vi "SignalReceiverCreat.vi"() -> (14 "SignalReceiver out":refnum<class "SignalReceiver.lvclass">, 15 "事件注册引用句柄":refnum<event-registration>, 19 "错误输出":errorcluster)   [LabVIEW 2020, in "ECU_Diagnose.lvlib" / "SignalReceiver.lvclass"]
uses:
  SignalReceiver.lvclass
  C:/Program Files (x86)/National Instruments/LabVIEW 2020/vi.lib/JKI/JKI SMO/SMO/SMO.lvclass
  Typedefs/PublicEvents--Cluster.ctl
  Typedefs/SetpointChanged--EventData--Cluster.ctl
  Typedefs/Data.ctl
  <vilib>/JKI/JKI SMO/SMO/Typedefs/Public Events.ctl
  <vilib>/JKI/JKI SMO/SMO/Typedefs/SMOState --Enum.ctl
  <vilib>/JKI/JKI SMO/SMO/Typedefs/Reserve State--Enum.ctl
  <vilib>/JKI/JKI SMO/SMO/SMO.lvclass/SMO.ctl
  <vilib>/JKI/JKI SMO/SMO/Private/ReftoDVR--SMO.vi
  <vilib>/JKI/JKI SMO/SMO/SMO.lvclass
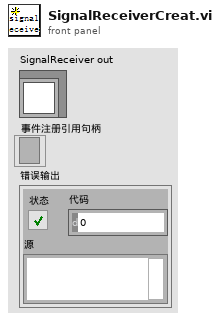
[diagram p1: front panel]
types:
  T1 = typedef "ECU_Diagnose.lvlib/SignalReceiver.lvclass/SignalArrySelecte.ctl" = cluster{"Port_No.":refnum<k21>, "XNET Signal":refnum<k21>[]}
  T2 = typedef "SMO.lvclass/Public Events.ctl" = cluster{"Error":refnum<user-event>, "State":refnum<user-event>, "Reserve State":refnum<user-event>}
  T3 = typedef "ECU_Diagnose.lvlib/SignalReceiver.lvclass/PublicEvents--Cluster.ctl" = cluster{"Setpoint Changed":refnum<user-event>, "Value Changed":refnum<user-event>}
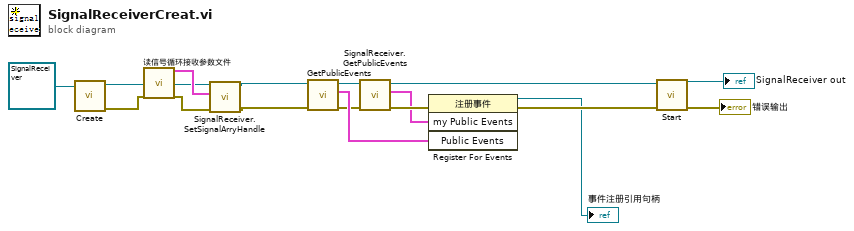
[diagram p0: block diagram]
diagram:
  n1 = call <vilib>:"Create.vi"("SMO"=refnum<class "SignalReceiver.lvclass"> refnum ("SMO.Template.lvclass")) -> ("error out"=w2:errorcluster, "SMO out"=w15:refnum<class "SignalReceiver.lvclass">)  [unwired: 8 in, 1 out]
  n2 = call "读信号循环接收参数文件.vi"("error in (no error)"=w2) -> ("SignalArryOut"=w17:T1, "error out"=w1:errorcluster)  [unwired: 17 in]
  n3 = call "SignalReceiver.SetSignalArryHandle.vi"("error in (no error)"=w1, "SignalArrySelect"=w17, "SignalReceiver"=w15) -> ("error out"=w16:errorcluster, "SignalReceiver out"=w8:refnum<class "SignalReceiver.lvclass">)  [unwired: 7 in]
  n4 = call <vilib>:"GetPublicEvents.vi"("error in (no error)"=w16, "SMO"=w8) -> ("error out"=w11:errorcluster, "Public Events"=w14:T2, "SMO out"=w12:refnum<class "SignalReceiver.lvclass">)  [unwired: 7 in]
  n5 = call "SignalReceiver.GetPublicEvents.vi"("error in (no error)"=w11, "SignalReceiver"=w12) -> ("error out"=w13:errorcluster, "my Public Events"=w10:T3, "SignalReceiver out"=w7:refnum<class "SignalReceiver.lvclass">)  [unwired: 7 in]
  n6 = register-events(error in=w13, w10, w14) -> (reference out=→"事件注册引用句柄":refnum<event-registration>, error out=w6:errorcluster)  [unwired: 1 in]
  n7 = call <vilib>:"Start.vi"("error in (no error)"=w6, "SMO"=w7) -> ("error out"=→"错误输出":errorcluster, "SMO out"=→"SignalReceiver out":refnum<class "SignalReceiver.lvclass">)  [unwired: 8 in]
